vi "SubDataDyn_P.vi"(10 "cluster":T2, 11 "Cluster en entrée":T1) -> (2 "Chaîne":string, 3 "cluster de sortie":T1)   [LabVIEW 2020]
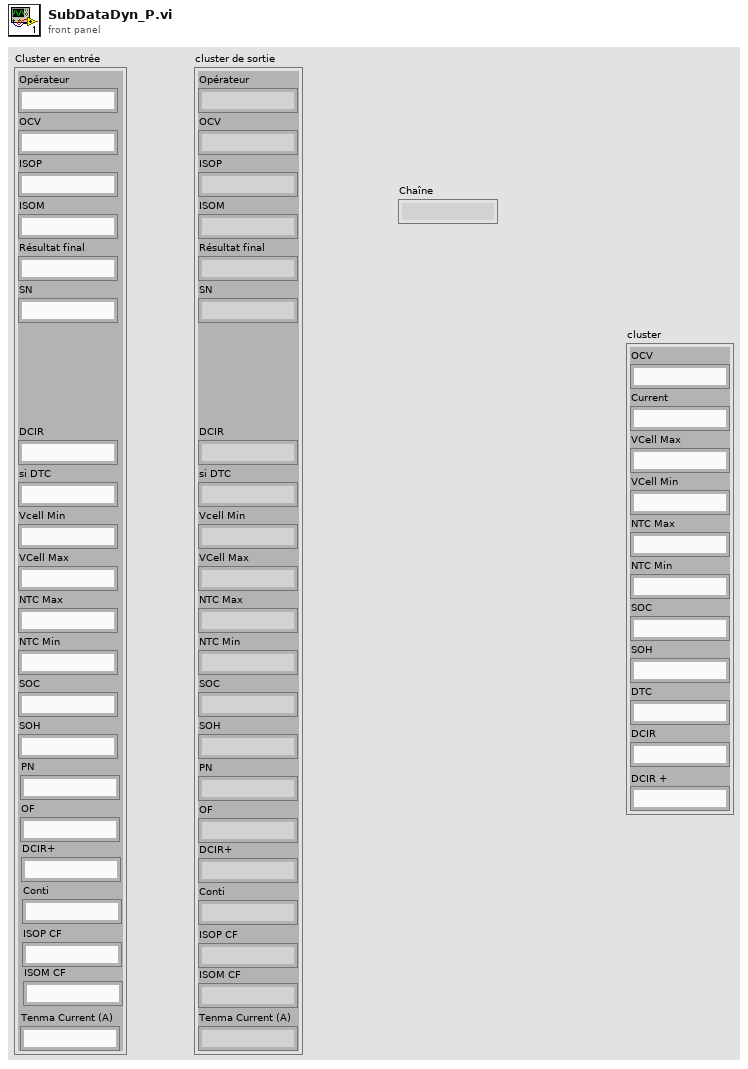
[diagram p1: front panel]
types:
  T1 = cluster{"Opérateur":string, "OCV":string, "ISOP":string, "ISOM":string, "Résultat final":string, "SN":string, "DCIR":string, "si DTC":string, "Vcell Min":string, "VCell Max":string, "NTC Max":string, "NTC Min":string, "SOC":string, "SOH":string, "PN":string, "OF":string, "DCIR+":string, "Conti":string, "ISOP CF":string, "ISOM CF":string, "Tenma Current (A)":string}
  T2 = cluster{"OCV":string, "Current":string, "VCell Max":string, "VCell Min":string, "NTC Max":string, "NTC Min":string, "SOC":string, "SOH":string, "DTC":string, "DCIR":string, "DCIR +":string}
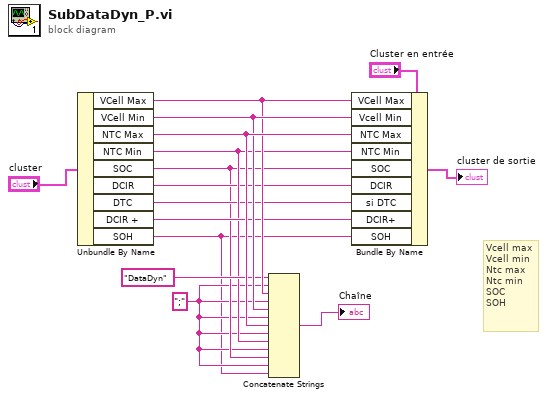
[diagram p0: block diagram]
diagram:
  w2 = ";" ("chaîne")
  # "Vcell max\nVcell min\nNtc max\nNtc min\nSOC\nSOH"
  n1 = Unbundle By Name("cluster") -> ("VCell Max"=w13:string, "VCell Min"=w14:string, "NTC Max"=w15:string, "NTC Min"=w6:string, "SOC"=w3:string, "DCIR"=w5:string, "DTC"=w4:string, "DCIR +"=w7:string, "SOH"=w1:string)
  n2 = Concatenate Strings("DataDyn" ("chaîne"), w2, w13, w2, w14, w2, w15, w2, w6, w2, w3, w2, w1) -> (→"Chaîne":string)
  n3 = Bundle By Name(cluster="Cluster en entrée", "VCell Max"=w13, "Vcell Min"=w14, "NTC Max"=w15, "NTC Min"=w6, "SOC"=w3, "DCIR"=w5, "si DTC"=w4, "DCIR+"=w7, "SOH"=w1) -> (→"cluster de sortie":T1)
